vi "TIFFStream Unique Filename.vi"(11 "Path in":path) -> (3 "Unique path out":path)   [LabVIEW 2018]
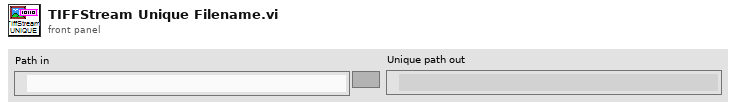
[diagram p1: front panel]
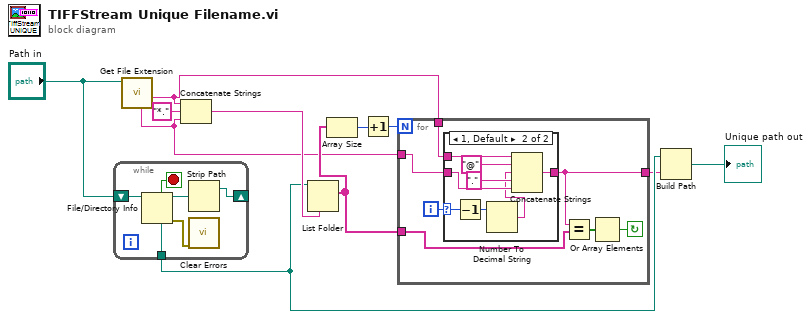
[diagram p0: block diagram]
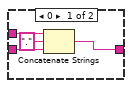
[diagram p2: hidden frame]
diagram:
  n1 = while {
    shift-right: [w15] -> _
    shift-left: "Path in" -> [w17]
    tunnel: [w13] -> w4
    stop <- w14 stop-if-true
    n2 = File/Directory Info(path=w17) -> (path out=w16:path, directory=w14:bool, error out=w12:errorcluster, resolved path=w13:path)  [unwired: 1 in, 3 out]
    n3 = Strip Path(path=w16) -> (stripped path=w15:path)  [unwired: 1 out]
    n4 = call <vilib>:"Clear Errors.vi"("error in (no error)"=w12) -> ()  [unwired: 5 in, 2 out]
  }
  n5 = call <vilib>:"Get File Extension.vi"("file"="Path in") -> ("filename without extension"=w6:string, "unmodified file extension"=w5:string)  [unwired: 6 in, 3 out]
  n6 = Concatenate Strings(w6, "*." ("string"), w5) -> (w9:string)
  n7 = List Folder(path=w4, pattern=w9) -> (filenames=w7:string[])  [unwired: 2 in, 3 out]
  n8 = Array Size(array=w7) -> (size(s)=w8:i32)
  n9 = Increment(x=w8) -> (x+1=w3:i32)
  n10 = for {
    N: w3 -> [_]
    tunnel: w7 -> [w21]
    tunnel: w6 -> [w24]
    tunnel: w5 -> [w22]
    tunnel: [w18] -> w2
    i -> [w23]
    stop <- w19 continue-if-true
    n11 = case shown="1, Default" w23 {
      selector: w23 -> [_ w31]
      tunnel: w24 -> [w28 w36]
      tunnel: w22 -> [w27 w35]
      tunnel: [w25 w29] -> w18
      frame 0 {
        n12 = Concatenate Strings(w28, "." ("string"), w27) -> (w25:string)
      }
      frame 1, Default {
        n13 = Decrement(x=w31) -> (x-1=w32:i32)
        n14 = Number To Decimal String(number=w32) -> (decimal integer string=w30:string)  [unwired: 1 in]
        n15 = Concatenate Strings(w36, "@" ("string"), w30, "." ("string"), w35) -> (w29:string)
      }
    }
    n16 = Equal?(x=w18, y=w21) -> (x = y?=w20:bool[])
    n17 = Or Array Elements(Boolean array=w20) -> (logical OR=w19:bool)
  }
  n18 = Build Path(base path=w4, name or relative path=w2) -> (appended path=→"Unique path out":path)
